vi "CH_LM Config Statistics Display Item.vi"(0 "Meter Index":i32, 2 "Display Item List":T1[](array[typedef]), 5 "error in (no error)":errorcluster, 7 "Timeout / ms (3000)":i32=3000, 8 "Action (query)":bool, 9 "Lock Timeout / ms (1000)":i32=1000) -> (11 "Lock timed out":bool, 14 "Meter Index":i32, 16 "Display Item List":T1[](array[typedef]), 19 "error out":errorcluster)   [LabVIEW 2012, in "CH_LM.lvlib"]
doc: "This command will select the statistics display items, which takes effect at the end of the current statistical batch. The data argument is a comma-separated list of one or more tokens shown below. At least one token must be specified. The tokens may be specified in any order. Duplicated tokens will be ignored. Error 101 will be raised if the list length exceeds 10 entries.\n\nThe Greenbuster UI Specification specifies the order and layout of statistics display items. One or more display items may be selected but only the first six list items will be displayed. The query will return all selected tokens including non-displayed tokens following the order stated in the reply list below.\n\n<B>Attention:</B> DOSE and MISSed will not be accepted on the TO version. They will be accepted on the TOP version."
uses:
  CH_LM.lvlib
  CH_LM Statistics Display Item.ctl
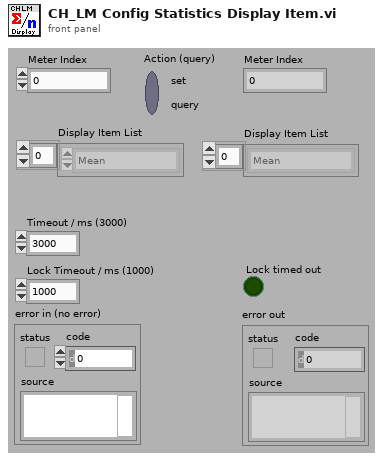
[diagram p1: front panel]
types:
  T1 = typedef "CH_LM.lvlib/CH_LM Statistics Display Item.ctl" = enum16{"Mean", "Minimum", "Maximum", "Standard Deviation", "1 Sigma", "2 Sigma", "3 Sigma", "Range", "Dose", "Missed"}
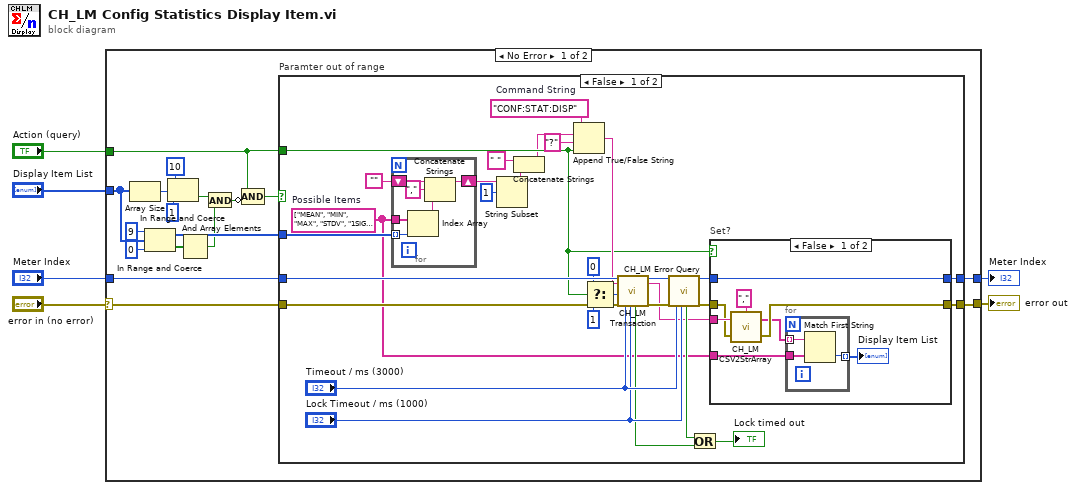
[diagram p0: block diagram]
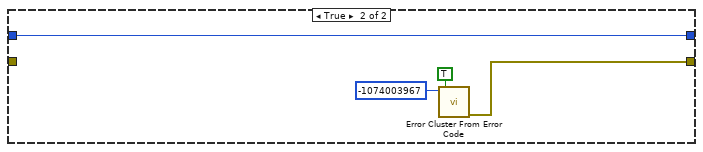
[diagram p3: hidden frame]
diagram:
  n1 = case shown="No Error" "error in (no error)" {
    selector: "error in (no error)" -> [w23 w77]
    tunnel: [w21 w77] -> w6
    tunnel: "Meter Index" -> [w22 w76]
    tunnel: [w20 w76] -> w3
    tunnel: "Action (query)" -> [w19 _]
    tunnel: "Display Item List" -> [w12 _]
    frame No Error {
      n2 = Array Size(array=w12) -> (size(s)=w17:i32)
      n3 = In Range and Coerce(upper limit=9, x=w12, lower limit=0) -> (coerced(x)=w11:i32[], In Range?=w10:bool[])
      n4 = In Range and Coerce(upper limit=10, x=w17, lower limit=1) -> (In Range?=w8:bool)  [unwired: 1 out]
      n5 = And Array Elements(Boolean array=w10) -> (logical AND=w9:bool)
      n6 = And(x=w8, y=w9) -> (x .and. y?=w7:bool)
      n7 = Compound Arithmetic op=AND(w19, invert w7) -> (w18:bool)
      n8 = case "Paramter out of range" shown="False" w18 {
        tunnel: w23 -> [w52 _]
        tunnel: w22 -> [w51 w74]
        tunnel: [w32 w73] -> w21
        tunnel: [w30 w74] -> w20
        tunnel: w19 -> [w35 _]
        tunnel: w11 -> [w36 _]
        frame False {
          w27 = string[] ["MEAN", "MIN", "MAX", "STDV", "1SIG", "2SIG", "3SIG", "RANG", "DOSE", "MISS"]  # Possible Items
          w43 = "CONF:STAT:DISP"  # Command String
          n9 = for {
            tunnel: w36 -> [w70] mode=indexing
            tunnel: w27 -> [w71]
            shift-right: [w68] -> w29
            shift-left: "" -> [w69]
            n10 = Index Array(array=w71, index=w70) -> (element=w67:string)
            n11 = Concatenate Strings(w69, "," ("string"), w67) -> (w68:string)
          }
          n12 = String Subset(string=w29, offset (0)=1) -> (substring=w26:string)  [unwired: 1 out]
          n13 = Concatenate Strings(" " ("string"), w26) -> (w24:string)
          n14 = Append True/False String(1:w35, 2:"?" ("false string"), 3:w24, 4:w43) -> (0:w41:string)
          n15 = Select(t=0, s=w35, f=1) -> (s? t:f=w39:i32)
          n16 = call "CH_LM Transaction.vi"("Meter Index"=w51, "Command String"=w41, "NofStrings (-1:all)"=w39, "error in (no error)"=w52, "Timeout / ms (3000)"="Timeout / ms (3000)", "Lock Timeout / ms (1000)"="Lock Timeout / ms (1000)") -> ("Lock timed out"=w45:bool, "Meter Index"=w48:i32, "Response"=w34:string, "error out"=w47:errorcluster)  [unwired: 10 out]
          n17 = call "CH_LM Error Query.vi"("Meter Index"=w48, "error in (no error)"=w47, "Timeout / ms (3000)"="Timeout / ms (3000)", "Lock Timeout / ms (1000)"="Lock Timeout / ms (1000)") -> ("Lock timed out"=w46:bool, "Meter Index"=w31:i32, "error out"=w33:errorcluster)  [unwired: 13 out]
          n18 = Or(x=w46, y=w45) -> (x .or. y?=→"Lock timed out":bool)
          n19 = case "Set?" shown="False" w35 {
            tunnel: w34 -> [w59 _]
            tunnel: w33 -> [w58 w64]
            tunnel: [w57 w64] -> w32
            tunnel: w31 -> [w56 w65]
            tunnel: [w56 w65] -> w30
            tunnel: w27 -> [w53 _]
            frame False {
              n20 = call "CH_LM CSV2StrArray.vi"("error in (no error)"=w58, "CSL"=w59, "Separator (,)"=",") -> ("error out"=w57:errorcluster, "Strings"=w55:string[])
              n21 = for {
                tunnel: w55 -> [w63] mode=indexing
                tunnel: w53 -> [w62]
                tunnel: [w61] -> w54 mode=indexing
                n22 = Match First String(2:w62, 3:w63) -> (0:w61:i32)  [unwired: 1 out]
              }
              "Display Item List" <- w54
            }
            frame True {
            }
          }
        }
        frame True {
          n23 = call <vilib>:"Error Cluster From Error Code.vi"("show call chain? (False)"=TRUE, "error code (0)"=-1074003967) -> ("error out"=w73:errorcluster)  [unwired: 1 in, 6 out]
        }
      }
    }
    frame Error {
    }
  }
  "error out" <- w6
  "Meter Index" <- w3
